vi "kbSpeedControl.vi"() -> ()   [LabVIEW 2019]
uses:
  <vilib>/Utility/inputDevices.llb/keyboardAcquire.vi
  <vilib>/Utility/inputDevices.llb/closeKeyboard.vi
panel:
  out "2keySpeed":i8
  out "speed":i8(slide) scale=-100.0..100.0
  out "keys pressed":T1(array[ring])
  in  "Stop Button":bool
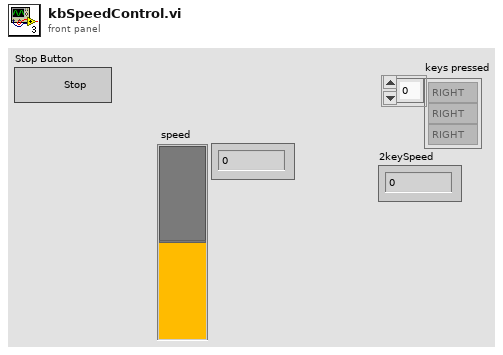
[diagram p1: front panel]
types:
  T1 = enum16{"0", "1", "2", "3", "4", "5", "6", "7", "8", "9", "A", "B", "C", "D", "E", "F", "G", "H", "I", "J", "K", "L", "M", "N", "O", "P", "Q", "R", "S", "T", "U", "V", "W", "X", "Y", "Z", "F1", "F2", "F3", "F4", "F5", "F6", "F7", "F8", "F9", "F10", "F11", "F12", "F13", "F14", "F15", "ADD", "BACK", "BACKSLASH", "CAPITAL", "COMMA", "DECIMAL", "DELETE", "DIVIDE", "DOWN", "END", "EQUALS", "ESCAPE", "GRAVE (`)", "HOME", "INSERT", "LBRACKET", "LCONTROL", "LEFT", "L ALT", "LSHIFT", "LWIN", "MINUS", "MULTIPLY", "NEXT", "NUMLOCK", "NUMPAD_0", "NUMPAD_1", "NUMPAD_2", "NUMPAD_3", "NUMPAD_4", "NUMPAD_5", "NUMPAD_6", "NUMPAD_7", "NUMPAD_8", "NUMPAD_9", "PAUSE", "PERIOD", "PRIOR (PG UP)", "RBRACKET", "RCONTROL", "RETURN", "RIGHT", "R ALT", "RSHIFT", "RWIN", "SCROLL", "SEMICOLON", "SLASH", "SPACE", "SUBTRACT", "TAB", "UP", "ENTER (num pad)", "' (quote)"}[]
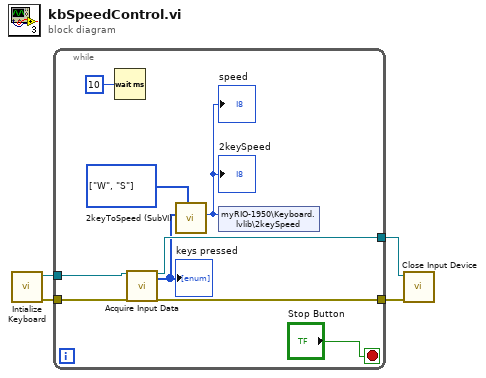
[diagram p0: block diagram]
diagram:
  n1 = call <vilib>:"Intialize Keyboard.vi"() -> ("error out"=w4:errorcluster, "device ID"=w2:refnum<k1>)  [unwired: 10 in]
  n2 = while {
    tunnel: w4 -> [w13]
    tunnel: [w12] -> w3
    tunnel: w2 -> [w11]
    tunnel: [w10] -> w1
    stop <- "Stop Button" stop-if-true
    w7 = T1 [enum."W", enum."S"] items=["0", "1", "2", "3", "4", "5", "6", "7", "8", "9", "A", "B", "C", "D", "E", "F", "G", "H", "I", "J", "K", "L", "M", "N", "O", "P", "Q", "R", "S", "T", "U", "V", "W", "X", "Y", "Z", "F1", "F2", "F3", "F4", "F5", "F6", "F7", "F8", "F9", "F10", "F11", "F12", "F13", "F14", "F15", "ADD", "BACK", "BACKSLASH", "CAPITAL", "COMMA", "DECIMAL", "DELETE", "DIVIDE", "DOWN", "END", "EQUALS", "ESCAPE", "GRAVE (`)", "HOME", "INSERT", "LBRACKET", "LCONTROL", "LEFT", "L ALT", "LSHIFT", "LWIN", "MINUS", "MULTIPLY", "NEXT", "NUMLOCK", "NUMPAD_0", "NUMPAD_1", "NUMPAD_2", "NUMPAD_3", "NUMPAD_4", "NUMPAD_5", "NUMPAD_6", "NUMPAD_7", "NUMPAD_8", "NUMPAD_9", "PAUSE", "PERIOD", "PRIOR (PG UP)", "RBRACKET", "RCONTROL", "RETURN", "RIGHT", "R ALT", "RSHIFT", "RWIN", "SCROLL", "SEMICOLON", "SLASH", "SPACE", "SUBTRACT", "TAB", "UP", "ENTER (num pad)", "' (quote)"] ("element")
    n3 = Wait (ms)(milliseconds to wait=u32 10) -> ()  [unwired: 1 out]
    n4 = call-poly <vilib>:"Acquire Input Data.vi"("device ID"=w11, "error in (no error)"=w13) -> ("device ID"=w10:refnum<k1>, "keys pressed"=w6:T1, "error out"=w12:errorcluster)  [unwired: 15 in]
    "keys pressed" <- w6
    n5 = call "2keyToSpeed (SubVI).vi"("key [+, -]"=w7, "keys pressed"=w6) -> ("2keySpeed"=w5:i8)  [unwired: 9 in]
    "speed" <- w5
    "2keySpeed" <- w5
    n6 = shared-variable "myRIO-1950\\Keyboard.lvlib\\2keySpeed"(w5) -> ()  [unwired: 1 in, 1 out]
  }
  n7 = call-poly <vilib>:"Close Input Device.vi"("error in (no error)"=w3, "device ID"=w1) -> ()  [unwired: 8 in, 1 out]
